vi "Parse Address Tree.vi"(8 "error in":errorcluster, 11 "Address Selection":string) -> (0 "error out":errorcluster, 3 "Address Parsed Tree":T1)   [LabVIEW 2023, in "J1939 Workspace Shared.lvlib"]
uses:
  J1939 Workspace Shared.lvlib
  Types/Address Parse Tree Cluster.ctl
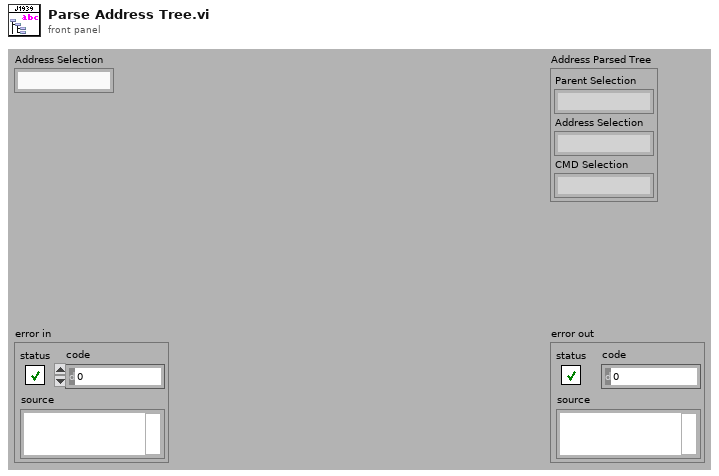
[diagram p1: front panel]
types:
  T1 = typedef "J1939 Workspace Shared.lvlib/Address Parse Tree Cluster.ctl" = cluster{"Parent Selection":string, "Address Selection":string, "CMD Selection":string}
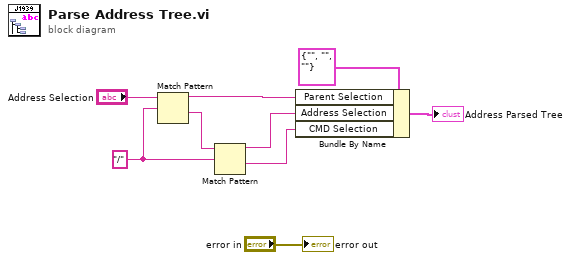
[diagram p0: block diagram]
diagram:
  w8 = "/" ("regular expression")
  n1 = Match Pattern(string="Address Selection", regular expression=w8) -> (before substring=w6:string, after substring=w7:string)  [unwired: 1 in, 2 out]
  n2 = Match Pattern(string=w7, regular expression=w8) -> (before substring=w5:string, after substring=w4:string)  [unwired: 1 in, 2 out]
  n3 = Bundle By Name(cluster=T1 {"Parent Selection"="", "Address Selection"="", "CMD Selection"=""} ("output cluster"), "Parent Selection"=w6, "Address Selection"=w5, "CMD Selection"=w4) -> (→"Address Parsed Tree":T1)
  "error out" <- "error in"
